vi "Recursive file list.vi"(8 "error in (no error)":errorcluster, 10 "Path":string, 11 "SCP File Transfer in":refnum<class "SCP File Transfer.lvclass">) -> (0 "error out":errorcluster, 1 "Files":string[](array[string]), 2 "Directories":string[](array[string]), 3 "SCP File Transfer out":refnum<class "SCP File Transfer.lvclass">)   [LabVIEW 2013, in "PL Framework Configuration Tool.lvlib" / "SCP File Transfer.lvclass"]
doc: "Returns an array of all directories and files located within the directory at \"Path\". It does not return the directory at \"Path\" in the array of directories.\n\nIf \"Continue on error?\" is false, the VI will immediately stop at the error, returning the directories and files found up until that point. If true, the VI will ignore errors, returning all directories and files that didn't encounter an error. In both cases, if an error occurs, that error is returned."
uses:
  SCP File Transfer.lvclass
  <vilib>/NI/RT Management/classes/File Transfer Behavior/File Transfer Behavior.lvclass
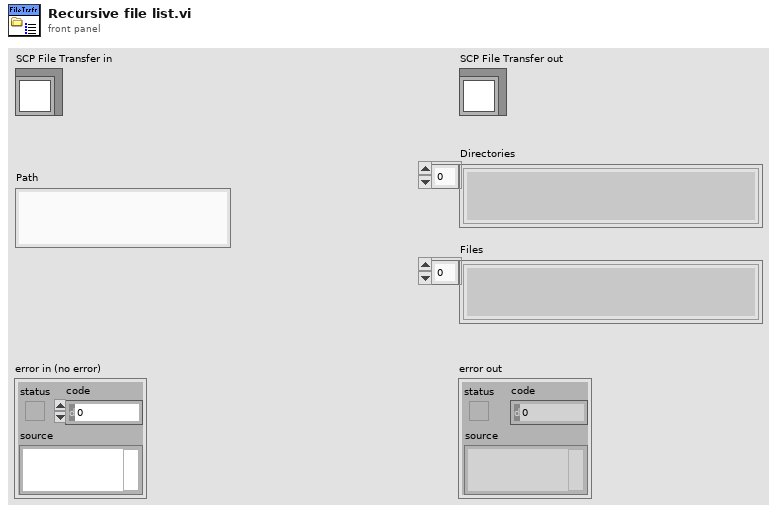
[diagram p1: front panel]
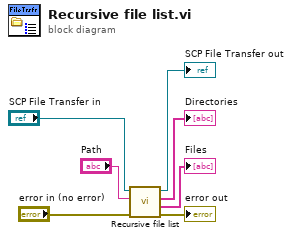
[diagram p0: block diagram]
diagram:
  n1 = call-parent "Recursive file list.vi"("error in (no error)"="error in (no error)", "Path"="Path", "File Transfer Behavior in"="SCP File Transfer in") -> ("error out"=→"error out":errorcluster, "Files"=→"Files":string[], "Directories"=→"Directories":string[], "File Transfer Behavior out"=→"SCP File Transfer out":refnum<class "SCP File Transfer.lvclass">)  [unwired: 5 in]
